vi "transmitSAL.vi"(8 "error in (no error)":errorcluster, 11 "Model in":refnum<class "Model.lvclass">) -> (0 "error out":errorcluster, 3 "Model out":refnum<class "Model.lvclass">)   [LabVIEW 2016, in "Model.lvclass"]
uses:
  Model.lvclass
  Model.lvclass/Model.ctl
  Publisher/Publisher.lvclass/Publisher.ctl
  Communicator/M1M3SAL/M1M3SAL.lvclass/M1M3SAL.ctl
  Communicator/M1M3SAL/write.vi
  Publisher/Publisher.lvclass
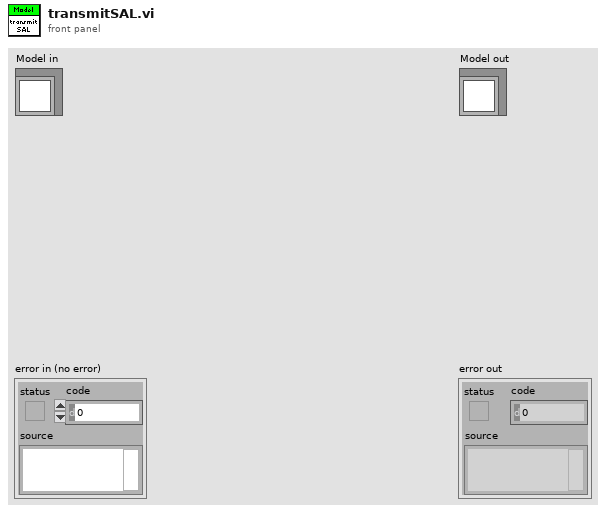
[diagram p1: front panel]
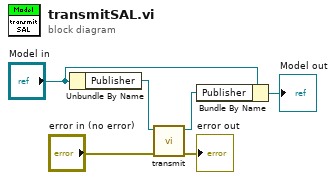
[diagram p0: block diagram]
diagram:
  n1 = Unbundle By Name("Model in") -> ("Publisher"=w4:refnum<class "Publisher.lvclass">)
  n2 = call "transmit.vi"("error in (no error)"="error in (no error)", "Publisher in"=w4) -> ("error out"=→"error out":errorcluster, "Publisher out"=w3:refnum<class "Publisher.lvclass">)  [unwired: 8 in]
  n3 = Bundle By Name(cluster="Model in", "Publisher"=w3) -> (→"Model out":refnum<class "Model.lvclass">)
